vi "control.vi"() -> ()   [LabVIEW 2016]
uses:
  Dynamixel Motor/Public/Motor Operation/Low Level/Baud Setting.ctl
  Program Files (x86)/National Instruments/LabVIEW 2016/examples/Data Communication/Protocols/TCP/TCP Multiple Connections/controls/TCP Multiple Connections State.ctl
  Program Files (x86)/National Instruments/LabVIEW 2016/examples/Data Communication/Protocols/TCP/TCP Multiple Connections/controls/TCP Multiple Connections Data.ctl
  Controller Output.vi
  Dynamixel Motor/Dynamixel Motor.lvlib
panel:
  out "# of Connections 4":i32
  out "# of Connections 3":i32
  out "불리언":bool
  out "불리언 3":bool
  out "# of Connections 2":i32
  out "불리언 2":bool=TRUE
  out "# of Connections":i32
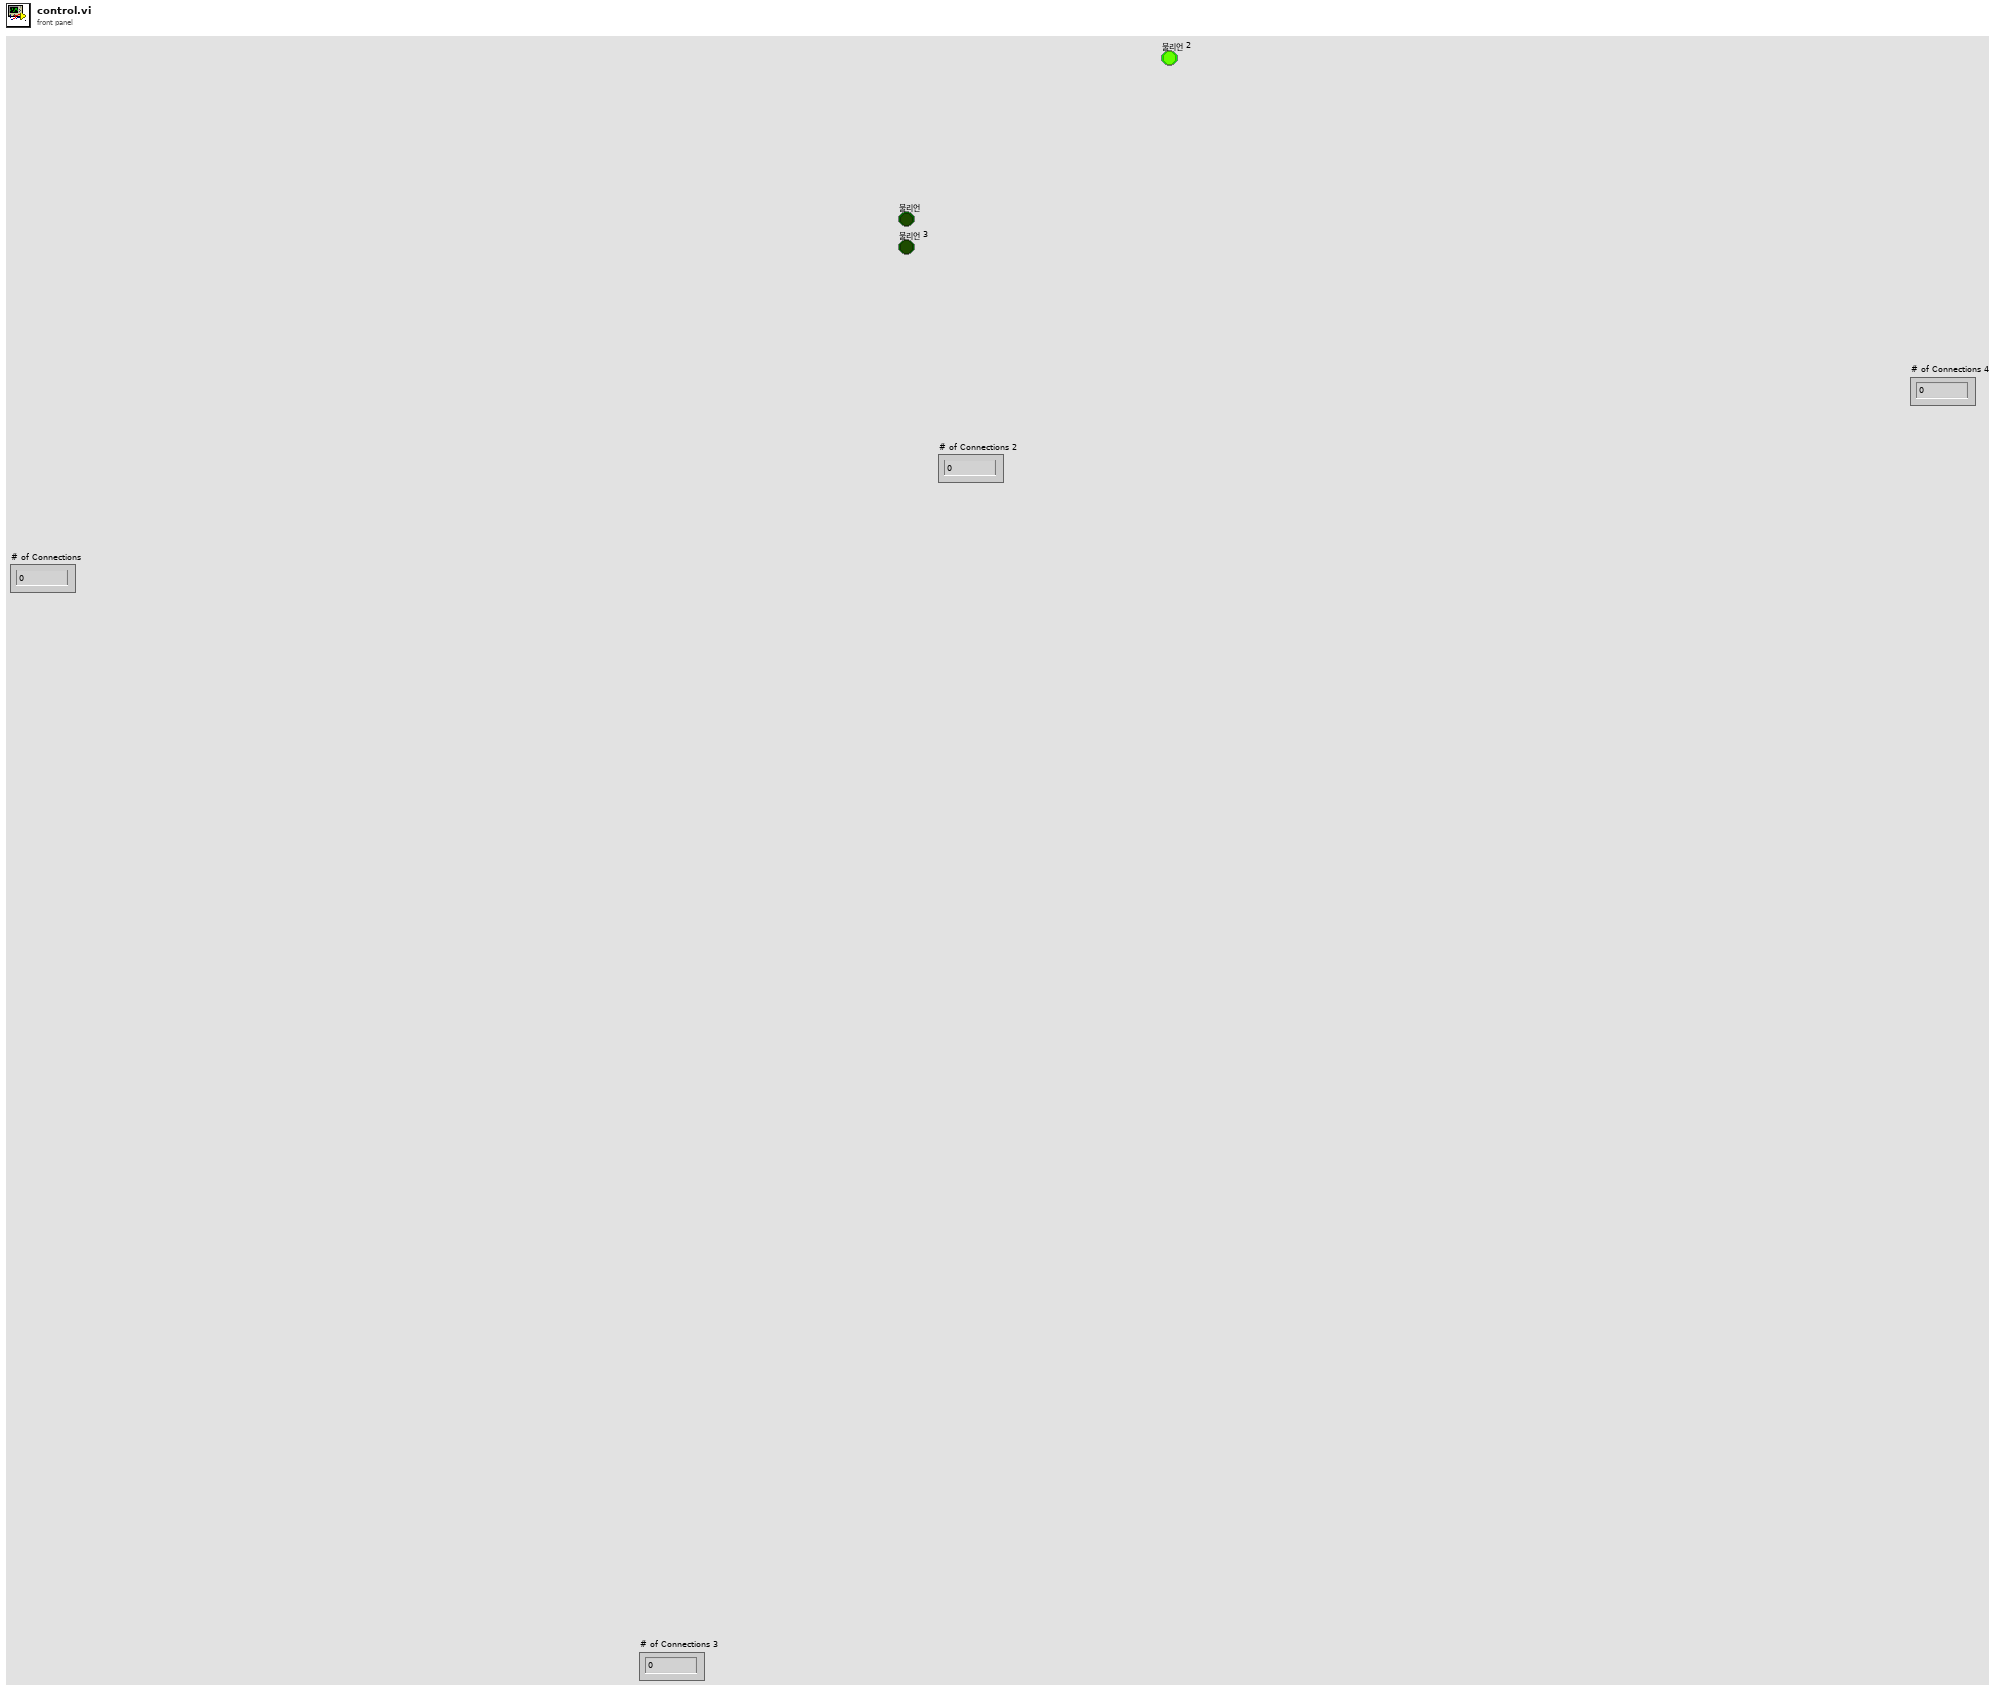
[diagram p1: front panel]
types:
  T1 = typedef "TCP Multiple Connections Data.ctl" = cluster{"Clients":refnum<k5>[], "Listener":refnum<k5>}
  T2 = typedef "TCP Multiple Connections State.ctl" = enum16{"Initialize", "Status Check", "Send Data", "Stop"}
  T3 = typedef "Dynamixel Motor.lvlib/Baud Setting.ctl" = u8
  T4 = typedef "YSH_XBOX360_joystick.ctl" = cluster{"RR":bool, "RL":bool, "RD":bool, "RU":bool, "LR":bool, "LL":bool, "LD":bool, "LU":bool, "Back":bool, "Start":bool, "DPad":dbl, "D Pad":cluster{"0":bool, "45":bool, "90":bool, "135":bool, "180":bool, "215":bool, "270":bool, "315":bool}, "A":bool, "B":bool, "X":bool, "Y":bool, "LB":bool, "RB":bool, "LT":bool, "RT":bool, "Left Joy Push":bool, "Right Joy Push":bool, "Z axis - LT~RT":i32, "Joy1 X-axis":i32, "Joy2 X-axis":i32, "Joy2 Y-axis":i32, "Joy1 Y-axis":i32}
  T5 = enum16{"big-endian, network order", "native, host order", "little-endian"}
  T6 = cluster{"lx":sgl, "ly":sgl, "sla":sgl, "sll":sgl, "rx":sgl, "ry":sgl, "sra":sgl, "srl":sgl, "tl":sgl, "tr":sgl, "bup":sgl, "bdn":sgl, "bl":sgl, "br":sgl, "ba":sgl, "bb":sgl, "bx":sgl, "by":sgl, "back":sgl, "start":sgl, "ls":sgl, "rs":sgl, "lt":sgl, "rt":sgl}
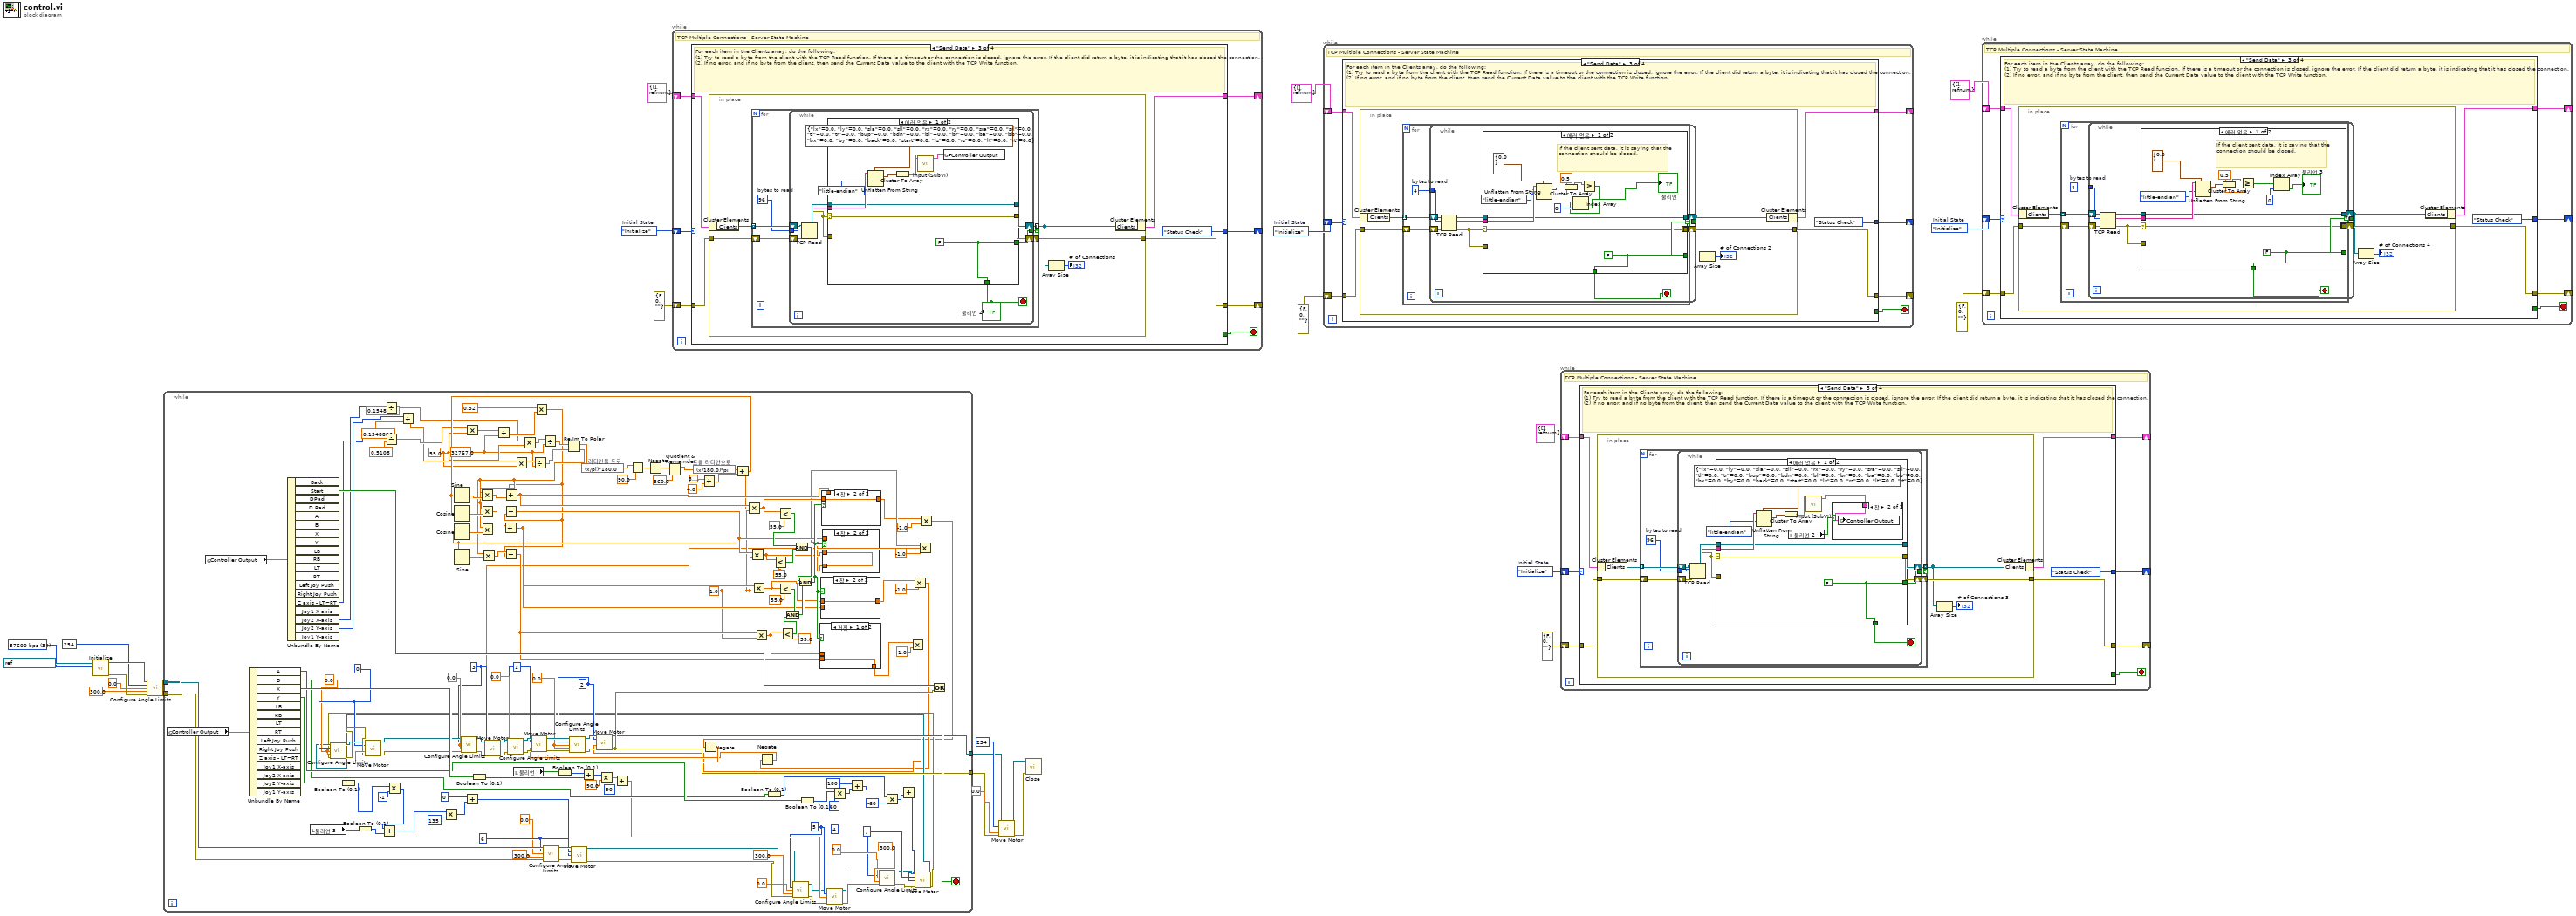
[diagram p0: block diagram]
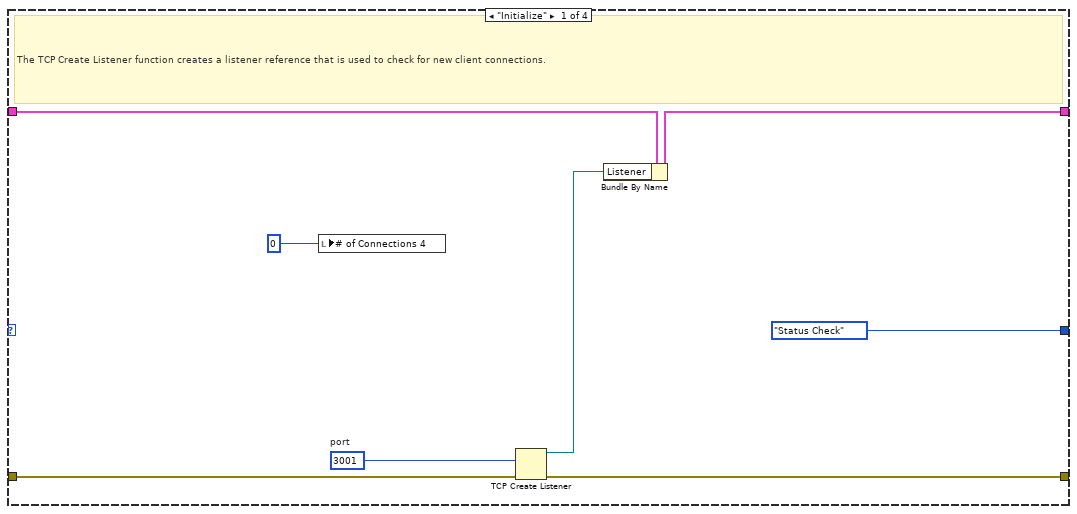
[diagram p2: hidden frame]
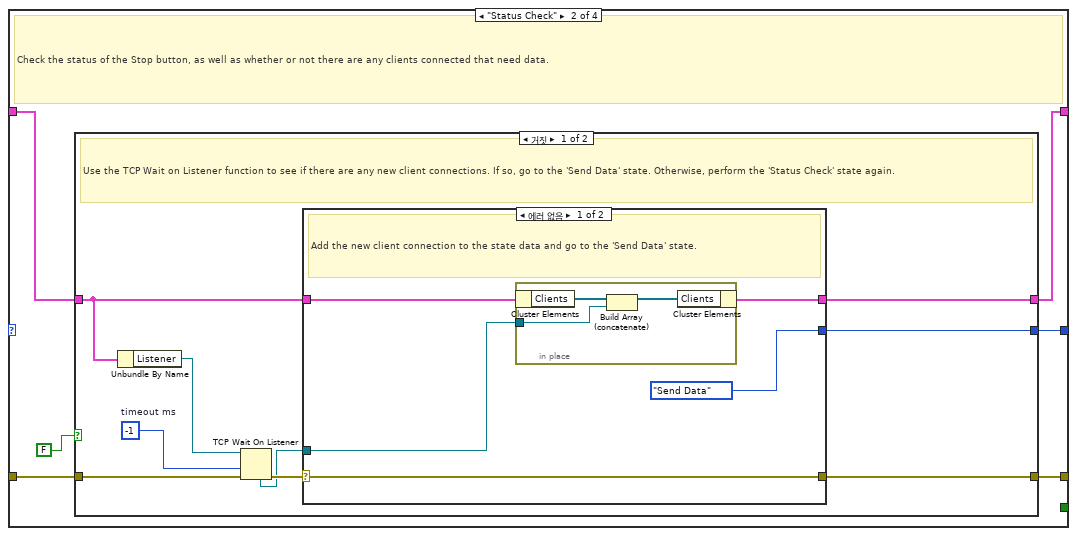
[diagram p3: hidden frame]
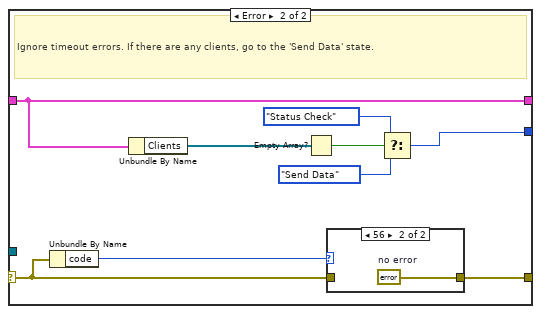
[diagram p4: hidden frame]
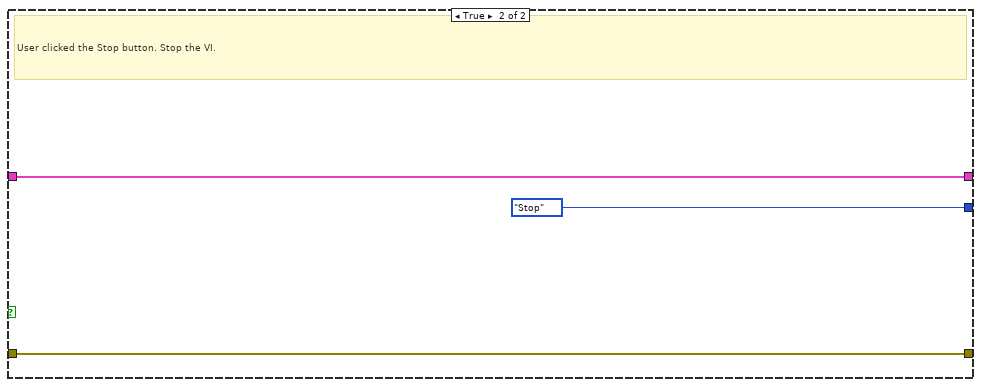
[diagram p6: hidden frame]
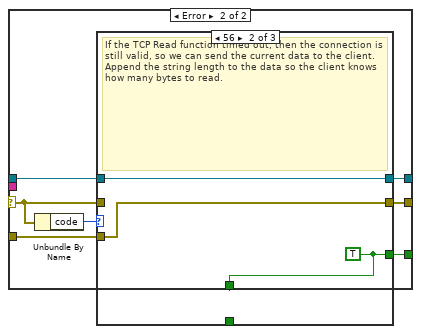
[diagram p7: hidden frame]
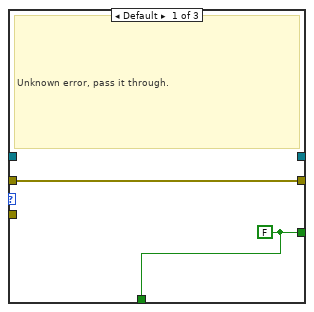
[diagram p8: hidden frame]
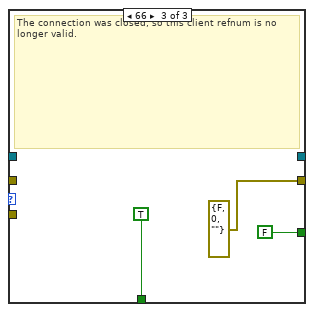
[diagram p9: hidden frame]
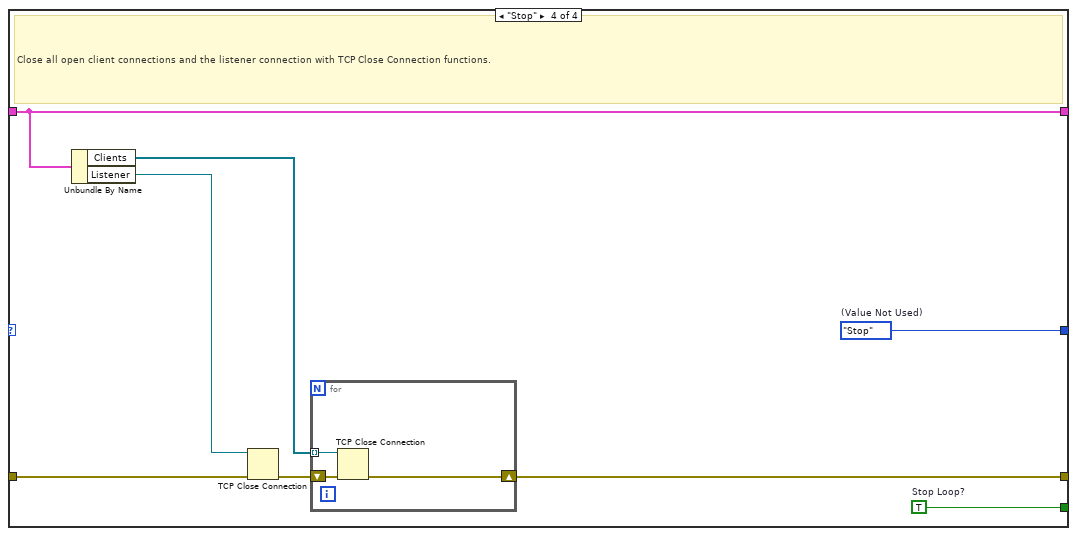
[diagram p10: hidden frame]
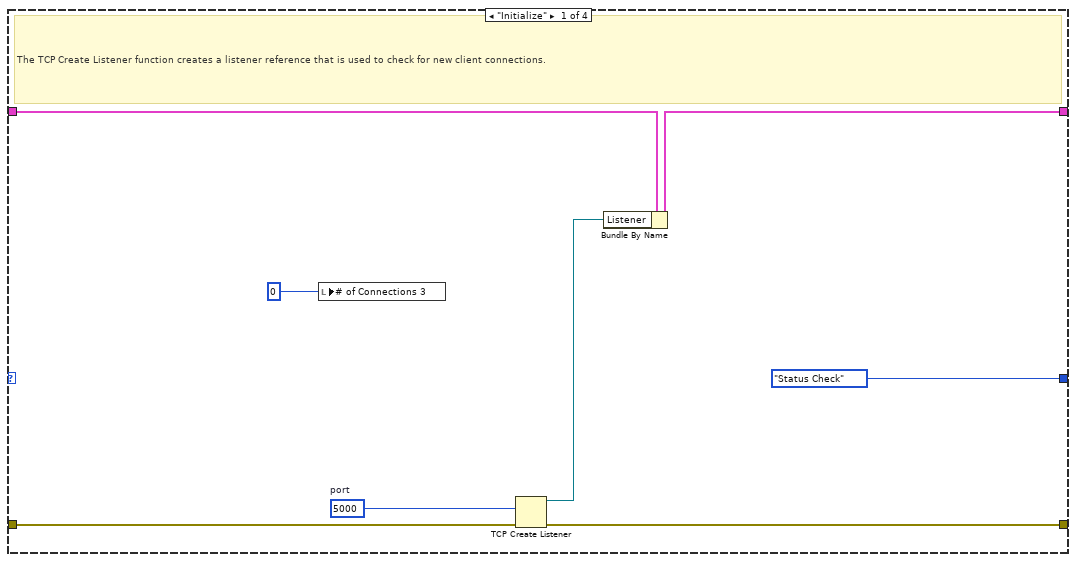
[diagram p15: hidden frame]
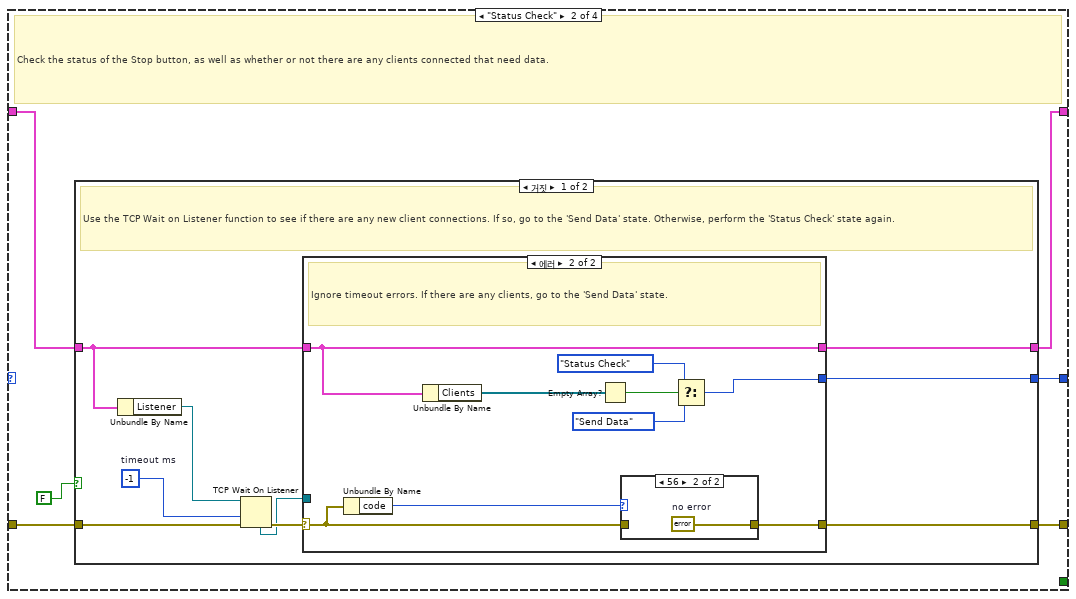
[diagram p16: hidden frame]
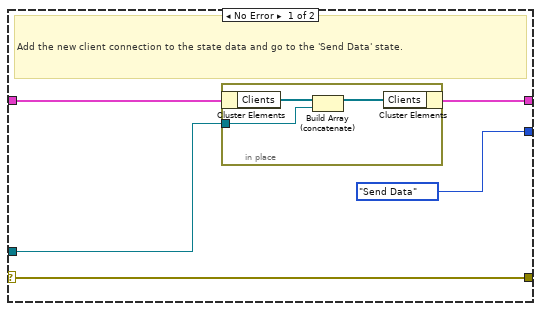
[diagram p17: hidden frame]
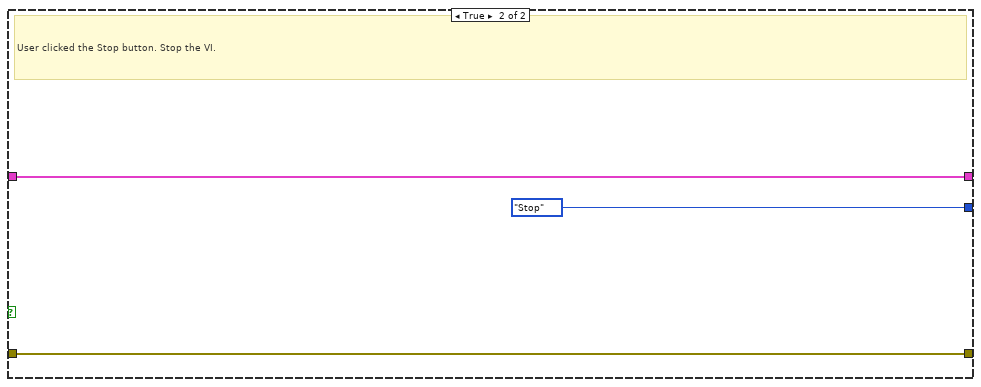
[diagram p19: hidden frame]
diagram:
  w3 = TCP_Multiple_Connections_State."Initialize"  # Initial State
  w17 = T3 34 items=["1,000,000 bps"=1, "500,000 bps"=3, "400,000 bps"=4, "250,000 bps"=7, "200,000 bps"=9, "115200 bps"=16, "57600 bps"=34, "19200 bps"=103, "9600 bps"=207] ("Baud rate (57600 bps) MX")
  w21 = TCP_Multiple_Connections_State."Initialize"  # Initial State
  w24 = TCP_Multiple_Connections_State."Initialize"  # Initial State
  w27 = TCP_Multiple_Connections_State."Initialize"  # Initial State
  n1 = call "Initialize.vi"("Baud rate (57600 bps)"=w17, "VISA resource name"=refnum<visa-resource-name> "ASRL3::INSTR") -> ("error out"=w13:errorcluster, "VISA resource name out"=w16:refnum<visa-resource-name>)  [unwired: 8 in]
  n2 = call "Configure Angle Limits.vi"("VISA resource name"=w16, "Motor ID (0)"=254, "Clockwise Angle Limit (0 deg)"=0.0, "Counter-Clockwise Angle Limit (300 deg)"=300.0, "error in (no error)"=w13) -> ("VISA resource name out"=w15:refnum<visa-resource-name>, "error out"=w14:errorcluster)  [unwired: 9 in]
  n3 = while {
    tunnel: w14 -> [w89]
    tunnel: [w100] -> w6
    tunnel: w15 -> [w91]
    tunnel: [w99] -> w7
    stop <- w126 stop-if-true
    w43 = 32767.0
    w44 = 55.0
    w87 = 6 ("Dynamixel ID AX sorting board 2")
    (unwired) 4 ("Dynamixel ID AX sorting board 2")
    w101 = u8 2 ("Motor ID4")
    w104 = u8 1 ("Motor ID3")
    w121 = u8 0 ("Motor ID1")
    w106 = u8 3 ("Motor ID2")
    w59 = 7 ("Dynamixel ID AX 문 개패 2")
    w49 = 5 ("Dynamixel ID AX sorting board 2")
    w92 = 1.0
    w113 = 0.0
    w105 = 0.0
    w102 = 0.0
    w120 = 0.0
    n4 = global read "Controller Output.vi" "Controller Output"() -> (w138:T4)
    n5 = global read "Controller Output.vi" "Controller Output"() -> (w142:T4)
    n6 = Unbundle By Name(w138) -> ("A"=w140:bool, "B"=w79:bool, "X"=w141:bool, "Y"=w81:bool)  [unwired: 11 out]
    n7 = Unbundle By Name(w142) -> ("Start"=w158:bool, "Z axis - LT~RT"=w71:i32, "Joy2 X-axis"=w73:i32, "Joy2 Y-axis"=w72:i32)  [unwired: 15 out]
    n8 = local read "불리언 3"() -> (w66:bool)
    n9 = Boolean To (0,1)(Boolean=w81) -> (0, 1=w41:i16)
    n10 = Boolean To (0,1)(Boolean=w66) -> (0, 1=w65:i16)
    n11 = Divide(x=w73, y=0.1548886) -> (x/y=w68:dbl)
    n12 = Divide(x=w71, y=0.5108) -> (x/y=w70:dbl)
    n13 = Multiply(x=w41, y=-1) -> (x*y=w40:i32)
    n14 = Add(x=w40, y=w65) -> (x+y=w63:i32)
    n15 = Divide(x=w72, y=0.1548886) -> (x/y=w69:dbl)
    n16 = Multiply(x=w63, y=135) -> (x*y=w83:i32)
    n17 = Multiply(x=w70, y=w44) -> (x*y=w181:dbl)
    n18 = Add(x=0, y=w83) -> (x+y=w82:i32)
    n19 = Boolean To (0,1)(Boolean=w141) -> (0, 1=w132:i16)
    n20 = Divide(x=w181, y=w43) -> (x/y=w97:dbl)
    n21 = Multiply(x=w69, y=w44) -> (x*y=w182:dbl)
    n22 = local read "불리언"() -> (w125:bool)
    n23 = Multiply(x=w68, y=w44) -> (x*y=w183:dbl)
    n24 = Divide(x=w182, y=w43) -> (x/y=w179:dbl)
    n25 = Multiply(x=0.32, y=w97) -> (x*y=w95:dbl)
    n26 = Divide(x=w183, y=w43) -> (x/y=w180:dbl)
    n27 = call "Configure Angle Limits.vi"("VISA resource name"=w91, "Motor ID (0)"=w87, "Clockwise Angle Limit (0 deg)"=0.0, "Counter-Clockwise Angle Limit (300 deg)"=300.0, "error in (no error)"=w89) -> ("VISA resource name out"=w90:refnum<visa-resource-name>, "error out"=w88:errorcluster)  [unwired: 9 in]
    n28 = Boolean To (0,1)(Boolean=w125) -> (0, 1=w131:i16)
    n29 = Re/Im To Polar(2:w179, 3:w180) -> (0:w178:dbl, 1:w163:dbl)
    n30 = call "Move Motor.vi"("VISA resource name"=w90, "Motor ID (0)"=w87, "Goal Position (180 deg)"=w82, "error in (no error)"=w88) -> ("VISA resource name out"=w45:refnum<visa-resource-name>, "error out"=w46:errorcluster)  [unwired: 10 in]
    n31 = Add(x=w131, y=w132) -> (x+y=w130:i16)
    n32 = expression code="(x/pi)*180.0" "라디안을 도로"(w178) -> (w177:dbl)
    n33 = Multiply(x=w130, y=90.0 ("sorting board 각도 input  2")) -> (x*y=w128:dbl)
    n34 = Add(x=w128, y=90) -> (x+y=w52:dbl)
    n35 = Subtract(x=w177, y=90.0) -> (x-y=w176:dbl)
    n36 = Negate(x=w176) -> (-x=w175:dbl)
    n37 = Quotient & Remainder(x=w175, y=360.0) -> (x-y*floor(x/y)=w172:dbl)  [unwired: 1 out]
    n38 = expression code="(x/180.0)*pi" "도를 라디안으로"(w172) -> (w171:dbl)
    n39 = Divide(x=3.141592653589793, y=4.0) -> (x/y=w168:dbl)
    n40 = Add(x=w171, y=w168) -> (x+y=w98:dbl)
    n41 = Sine(x=w98) -> (sin(x)=w167:dbl)
    n42 = Cosine(x=w98) -> (cos(x)=w166:dbl)
    n43 = Cosine(x=w98) -> (cos(x)=w165:dbl)
    n44 = Sine(x=w98) -> (sin(x)=w164:dbl)
    n45 = Multiply(x=w163, y=w167) -> (x*y=w161:dbl)
    n46 = Multiply(x=w163, y=w166) -> (x*y=w160:dbl)
    n47 = Multiply(x=w163, y=w165) -> (x*y=w162:dbl)
    n48 = Multiply(x=w163, y=w164) -> (x*y=w159:dbl)
    n49 = Add(x=w95, y=w162) -> (x+y=w135:dbl)
    n50 = Subtract(x=w160, y=w95) -> (x-y=w136:dbl)
    n51 = Subtract(x=w159, y=w95) -> (x-y=w134:dbl)
    n52 = Add(x=w95, y=w161) -> (x+y=w137:dbl)
    n53 = Multiply(x=w137, y=w92) -> (x*y=w156:dbl)
    n54 = Multiply(x=w136, y=w92) -> (x*y=w145:dbl)
    n55 = Multiply(x=w135, y=w92) -> (x*y=w144:dbl)
    n56 = Multiply(x=w134, y=w92) -> (x*y=w143:dbl)
    n57 = Boolean To (0,1)(Boolean=w79) -> (0, 1=w78:i16)
    n58 = Less?(x=w145, y=55.0) -> (x < y?=w149:bool)
    n59 = Less?(x=w156, y=55.0) -> (x < y?=w155:bool)
    n60 = Less?(x=w144, y=55.0) -> (x < y?=w150:bool)
    n61 = Less?(x=w143, y=55.0) -> (x < y?=w151:bool)
    n62 = And(x=w150, y=w151) -> (x .and. y?=w147:bool)
    n63 = call "Configure Angle Limits.vi"("VISA resource name"=w45, "Motor ID (0)"=w49, "Clockwise Angle Limit (0 deg)"=0.0, "Counter-Clockwise Angle Limit (300 deg)"=300.0, "error in (no error)"=w46) -> ("VISA resource name out"=w48:refnum<visa-resource-name>, "error out"=w47:errorcluster)  [unwired: 9 in]
    n64 = And(x=w155, y=w149) -> (x .and. y?=w148:bool)
    n65 = And(x=w148, y=w147) -> (x .and. y?=w146:bool)
    n66 = Boolean To (0,1)(Boolean=w140) -> (0, 1=w129:i16)
    n67 = case shown="거짓" w146 {
      tunnel: w143 -> [_ w187]
      tunnel: w134 -> [w186 _]
      tunnel: [w186 w187] -> w35
      frame False {
      }
      frame True {
      }
    }
    n68 = case shown="참" w146 {
      tunnel: w144 -> [_ w185]
      tunnel: [w184 w185] -> w33
      tunnel: w135 -> [w184 _]
      frame False {
      }
      frame True {
      }
    }
    n69 = case shown="참" w146 {
      tunnel: w156 -> [_ w191]
      tunnel: [w190 w191] -> w29
      tunnel: w137 -> [w190 _]
      frame False {
      }
      frame True {
      }
    }
    n70 = case shown="참" w146 {
      tunnel: w145 -> [_ w189]
      tunnel: w136 -> [w188 _]
      tunnel: [w188 w189] -> w30
      frame False {
      }
      frame True {
      }
    }
    n71 = call "Move Motor.vi"("VISA resource name"=w48, "Motor ID (0)"=w49, "Goal Position (180 deg)"=w52, "error in (no error)"=w47) -> ("VISA resource name out"=w54:refnum<visa-resource-name>, "error out"=w53:errorcluster)  [unwired: 10 in]
    n72 = Multiply(x=w129, y=60) -> (x*y=w93:i32)
    n73 = Add(x=180, y=w93) -> (x+y=w77:i32)
    n74 = call "Configure Angle Limits.vi"("VISA resource name"=w54, "Motor ID (0)"=w59, "Clockwise Angle Limit (0 deg)"=0.0, "Counter-Clockwise Angle Limit (300 deg)"=300.0, "error in (no error)"=w53) -> ("VISA resource name out"=w58:refnum<visa-resource-name>, "error out"=w60:errorcluster)  [unwired: 9 in]
    n75 = Multiply(x=w78, y=-60) -> (x*y=w76:i32)
    n76 = Add(x=w77, y=w76) -> (x+y=w57:i32)
    n77 = Multiply(x=w35, y=-1.0) -> (x*y=w34:dbl)
    n78 = Multiply(x=w33, y=-1.0) -> (x*y=w32:dbl)
    n79 = Negate(x=w32) -> (-x=w103:dbl)
    n80 = call "Move Motor.vi"("VISA resource name"=w58, "Motor ID (0)"=w59, "Goal Position (180 deg)"=w57, "error in (no error)"=w60) -> ("VISA resource name out"=w56:refnum<visa-resource-name>, "error out"=w55:errorcluster)  [unwired: 10 in]
    n81 = call "Configure Angle Limits.vi"("VISA resource name"=w56, "Motor ID (0)"=w121, "Clockwise Angle Limit (0 deg)"=w120, "Counter-Clockwise Angle Limit (300 deg)"=w120, "error in (no error)"=w55) -> ("VISA resource name out"=w122:refnum<visa-resource-name>, "error out"=w123:errorcluster)  [unwired: 9 in]
    n82 = Multiply(x=w30, y=-1.0) -> (x*y=w31:dbl)
    n83 = Multiply(x=w29, y=-1.0) -> (x*y=w28:dbl)
    n84 = Negate(x=w28) -> (-x=w124:dbl)
    n85 = call "Move Motor.vi"("VISA resource name"=w122, "Motor ID (0)"=w121, "Goal Speed (RPM)"=w124, "error in (no error)"=w123) -> ("VISA resource name out"=w107:refnum<visa-resource-name>, "error out"=w119:errorcluster)  [unwired: 10 in]
    n86 = call "Configure Angle Limits.vi"("VISA resource name"=w107, "Motor ID (0)"=w106, "Clockwise Angle Limit (0 deg)"=w113, "Counter-Clockwise Angle Limit (300 deg)"=w113, "error in (no error)"=w119) -> ("VISA resource name out"=w112:refnum<visa-resource-name>, "error out"=w114:errorcluster)  [unwired: 9 in]
    n87 = call "Move Motor.vi"("VISA resource name"=w112, "Motor ID (0)"=w106, "Goal Speed (RPM)"=w31, "error in (no error)"=w114) -> ("VISA resource name out"=w111:refnum<visa-resource-name>, "error out"=w115:errorcluster)  [unwired: 10 in]
    n88 = call "Configure Angle Limits.vi"("VISA resource name"=w111, "Motor ID (0)"=w104, "Clockwise Angle Limit (0 deg)"=w105, "Counter-Clockwise Angle Limit (300 deg)"=w105, "error in (no error)"=w115) -> ("VISA resource name out"=w110:refnum<visa-resource-name>, "error out"=w116:errorcluster)  [unwired: 9 in]
    n89 = call "Move Motor.vi"("VISA resource name"=w110, "Motor ID (0)"=w104, "Goal Speed (RPM)"=w103, "error in (no error)"=w116) -> ("VISA resource name out"=w109:refnum<visa-resource-name>, "error out"=w117:errorcluster)  [unwired: 10 in]
    n90 = call "Configure Angle Limits.vi"("VISA resource name"=w109, "Motor ID (0)"=w101, "Clockwise Angle Limit (0 deg)"=w102, "Counter-Clockwise Angle Limit (300 deg)"=w102, "error in (no error)"=w117) -> ("VISA resource name out"=w108:refnum<visa-resource-name>, "error out"=w118:errorcluster)  [unwired: 9 in]
    n91 = call "Move Motor.vi"("VISA resource name"=w108, "Motor ID (0)"=w101, "Goal Speed (RPM)"=w34, "error in (no error)"=w118) -> ("VISA resource name out"=w99:refnum<visa-resource-name>, "error out"=w100:errorcluster)  [unwired: 10 in]
    n92 = Or(x=w158, y=w100) -> (x .or. y?=w126:bool)
  }
  n93 = while {
    shift-right: [w197] -> _
    shift-left: w27 -> [w198]
    shift-right: [w195] -> _
    shift-left: T1 {"Clients"=[], "Listener"=refnum} ("Data") -> [w196]
    shift-right: [w193] -> _
    shift-left: errorcluster {"status"=FALSE, "code"=0, "source"=""} ("error constant") -> [w194]
    stop <- w192 stop-if-true
    # "TCP Multiple Connections - Server State Machine"
    n94 = case shown="\"Send Data\"" w198 {
      tunnel: [TCP_Multiple_Connections_State."Status Check" ("States") w212 TCP_Multiple_Connections_State."Status Check" ("States") w296] -> w197
      tunnel: [_ _ _ w303] -> w192
      tunnel: w196 -> [w204 w208 w246 w302]
      tunnel: [w203 w207 w245 w302] -> w195
      tunnel: w194 -> [w206 w211 w248 w301]
      tunnel: [w205 w210 w247 w299] -> w193
      frame "Initialize" {
        w201 = u16 4000  # port
        # "The TCP Create Listener function creates a listener reference that is used to check for new client connections."
        n95 = local write "# of Connections"(0 ("Number of Client Connections")) -> ()
        n96 = TCP Create Listener(8:w206, 10:w201) -> (0:w205:errorcluster, 3:w202:refnum<k5>)  [unwired: 4 out]
        n97 = Bundle By Name(cluster=w204, "Listener"=w202) -> (w203:T1)
      }
      frame "Status Check" {
        # "Check the status of the Stop button, as well as whether or not there are any clients connected that need data."
        n98 = case shown="거짓" FALSE ("Stop") {
          tunnel: [w221 TCP_Multiple_Connections_State."Stop" ("States")] -> w212
          tunnel: w211 -> [w220 w243]
          tunnel: [w213 w243] -> w210
          tunnel: w208 -> [w216 w242]
          tunnel: [w215 w242] -> w207
          frame False {
            w219 = -1  # timeout ms
            # "Use the TCP Wait on Listener function to see if there are any new client connections. If so, go to the 'Send Data' state. Otherwise, perform the 'Status Check' state again."
            n99 = Unbundle By Name(w216) -> ("Listener"=w214:refnum<k5>)
            n100 = TCP Wait On Listener(8:w220, 9:w219, 11:w214) -> (0:w218:errorcluster, 4:w217:refnum<k5>)  [unwired: 4 out]
            n101 = case shown="에러 없음" w218 {
              selector: w218 -> [w224 w238]
              tunnel: [TCP_Multiple_Connections_State."Send Data" ("States") w232] -> w221
              tunnel: w217 -> [w225 _]
              tunnel: w216 -> [w226 w235]
              tunnel: [w223 w235] -> w215
              tunnel: [w224 w236] -> w213
              frame No Error {
                # "Add the new client connection to the state data and go to the 'Send Data' state."
                n102 = in-place {
                  in-place-border: w225 -> [w227]
                  n103 = in-place-cluster #1(w226) -> ("Clients"=w229:refnum<k5>[])
                  n104 = Build Array (concatenate)(w229, w227) -> (w228:refnum<k5>[])
                  n105 = in-place-cluster #1("Clients"=w228) -> (w223:T1)
                }
              }
              frame Error {
                # "Ignore timeout errors. If there are any clients, go to the 'Send Data' state."
                n106 = Unbundle By Name(w238) -> ("code"=w237:i32)
                n107 = Unbundle By Name(w235) -> ("Clients"=w234:refnum<k5>[])
                n108 = Empty Array?(array=w234) -> (empty?=w233:bool)
                n109 = case shown="56" w237 {
                  tunnel: w238 -> [w239 _]
                  tunnel: [w239 w240] -> w236
                  frame Default {
                  }
                  frame 56 {
                    w240 = errorcluster {"status"=FALSE, "code"=0, "source"=""}  # no error
                  }
                }
                n110 = Select(t=TCP_Multiple_Connections_State."Status Check" ("States"), s=w233, f=TCP_Multiple_Connections_State."Send Data" ("States")) -> (s? t:f=w232:T2)
              }
            }
          }
          frame True {
            # "User clicked the Stop button. Stop the VI."
          }
        }
      }
      frame "Send Data" {
        # "For each item in the Clients array, do the following:\n(1) Try to read a byte from the client with the TCP Read function. If there is a timeout or the connection is closed, ignore the error. If the client did return a byte, it is indicating that it has closed the connection.\n(2) If no error, and if no byte from the client, then send the Current Data value to the client with the TCP Write function."
        n111 = in-place {
          in-place-border: w248 -> [w253]
          in-place-border: [w252] -> w247
          n112 = in-place-cluster #2(w246) -> ("Clients"=w250:refnum<k5>[])
          n113 = for {
            tunnel: w250 -> [w259] mode=indexing
            shift-right: [w255] -> w252
            shift-left: w253 -> [w254]
            tunnel: [w257] -> w249 mode=indexing if=w256
            w258 = 96  # bytes to read
            n114 = while {
              tunnel: w258 -> [w267]
              tunnel: [w264] -> w256
              shift-right: [w265] -> w257
              shift-left: w259 -> [w269]
              shift-right: [w261] -> w255
              shift-left: w254 -> [w263]
              stop <- w260 stop-if-true
              n115 = TCP Read(connection ID=w269, bytes to read=w267, error in (no error)=w263) -> (connection ID out=w268:refnum<k5>, data out=w266:string, error out=w262:errorcluster)  [unwired: 1 in, 1 out]
              n116 = case shown="에러 없음" w262 {
                selector: w262 -> [w271 w285]
                tunnel: w268 -> [w277 w284]
                tunnel: w266 -> [w278 _]
                tunnel: [w277 w282] -> w265
                tunnel: [w270 w283] -> w264
                tunnel: [w271 w281] -> w261
                tunnel: w262 -> [_ w280]
                tunnel: [w270 w279] -> w260
                frame No Error {
                  w270 = FALSE
                  # "If the client sent data, it is saying that the connection should be closed."
                  n117 = Unflatten From String(type=T6 {"lx"=0.0, "ly"=0.0, "sla"=0.0, "sll"=0.0, "rx"=0.0, "ry"=0.0, "sra"=0.0, "srl"=0.0, "tl"=0.0, "tr"=0.0, "bup"=0.0, "bdn"=0.0, "bl"=0.0, "br"=0.0, "ba"=0.0, "bb"=0.0, "bx"=0.0, "by"=0.0, "back"=0.0, "start"=0.0, "ls"=0.0, "rs"=0.0, "lt"=0.0, "rt"=0.0}, binary string=w278, byte order (0:big-endian, network order)=T5."little-endian") -> (value=w276:T6)  [unwired: 2 in, 2 out]
                  n118 = Cluster To Array(cluster=w276) -> (array=w273:sgl[])
                  n119 = call "input (SubVI).vi"("Controller_NUC"=w273) -> ("Controller Input"=w272:T4)  [unwired: 10 in]
                  n120 = global write "Controller Output.vi" "Controller Output"(w272) -> ()
                }
                frame Error {
                  # "Ignore connection closed and timeout errors"
                  n121 = Unbundle By Name(w285) -> ("code"=w286:i32)
                  n122 = case shown="66" w286 {
                    tunnel: w285 -> [w288 _ _]
                    tunnel: [w288 w290 errorcluster {"status"=FALSE, "code"=0, "source"=""} ("error constant")] -> w281
                    tunnel: w284 -> [_ w291 _]
                    tunnel: [w287 TRUE FALSE] -> w283
                    tunnel: [_ w291 _] -> w282
                    tunnel: w280 -> [_ w290 _]
                    tunnel: [w287 TRUE TRUE] -> w279
                    frame Default {
                      w287 = FALSE
                      # "Unknown error, pass it through."
                    }
                    frame 56 {
                      # "If the TCP Read function timed out, then the connection is still valid, so we can send the current data to the client. Append the string length to the data so the client knows how many bytes to read."
                    }
                    frame 66 {
                      # "The connection was closed, so this client refnum is no longer valid."
                    }
                  }
                }
              }
              "불리언 2" <- w260
            }
          }
          n123 = Array Size(array=w249) -> (size(s)=→"# of Connections":i32)
          n124 = in-place-cluster #2("Clients"=w249) -> (w245:T1)
        }
      }
      frame "Stop" {
        w296 = TCP_Multiple_Connections_State."Stop"  # (Value Not Used)
        w303 = TRUE  # Stop Loop?
        # "Close all open client connections and the listener connection with TCP Close Connection functions."
        n125 = Unbundle By Name(w302) -> ("Clients"=w300:refnum<k5>[], "Listener"=w297:refnum<k5>)
        n126 = TCP Close Connection(connection ID=w297, error in (no error)=w301) -> (error out=w298:errorcluster)  [unwired: 1 in, 1 out]
        n127 = for {
          shift-right: [w305] -> w299
          shift-left: w298 -> [w306]
          tunnel: w300 -> [w304] mode=indexing
          n128 = TCP Close Connection(connection ID=w304, error in (no error)=w306) -> (error out=w305:errorcluster)  [unwired: 1 in, 1 out]
        }
      }
    }
  }
  n129 = call "Move Motor.vi"("VISA resource name"=w7, "Motor ID (0)"=254, "Goal Speed (RPM)"=0.0, "error in (no error)"=w6) -> ("VISA resource name out"=w5:refnum<visa-resource-name>, "error out"=w4:errorcluster)  [unwired: 10 in]
  n130 = call "Close.vi"("error in (no error)"=w4, "VISA resource name"=w5) -> ()  [unwired: 9 in, 1 out]
  n131 = while {
    shift-right: [w312] -> _
    shift-left: w24 -> [w313]
    shift-right: [w310] -> _
    shift-left: T1 {"Clients"=[], "Listener"=refnum} ("Data") -> [w311]
    shift-right: [w308] -> _
    shift-left: errorcluster {"status"=FALSE, "code"=0, "source"=""} ("error constant") -> [w309]
    stop <- w307 stop-if-true
    # "TCP Multiple Connections - Server State Machine"
    n132 = case shown="\"Send Data\"" w313 {
      tunnel: [TCP_Multiple_Connections_State."Status Check" ("States") w327 TCP_Multiple_Connections_State."Status Check" ("States") w413] -> w312
      tunnel: [_ _ _ w420] -> w307
      tunnel: w311 -> [w319 w323 w361 w419]
      tunnel: [w318 w322 w360 w419] -> w310
      tunnel: w309 -> [w321 w326 w363 w418]
      tunnel: [w320 w325 w362 w416] -> w308
      frame "Initialize" {
        w316 = u16 3000  # port
        # "The TCP Create Listener function creates a listener reference that is used to check for new client connections."
        n133 = local write "# of Connections 2"(0 ("Number of Client Connections")) -> ()
        n134 = TCP Create Listener(8:w321, 10:w316) -> (0:w320:errorcluster, 3:w317:refnum<k5>)  [unwired: 4 out]
        n135 = Bundle By Name(cluster=w319, "Listener"=w317) -> (w318:T1)
      }
      frame "Status Check" {
        # "Check the status of the Stop button, as well as whether or not there are any clients connected that need data."
        n136 = case shown="거짓" FALSE ("Stop 2") {
          tunnel: [w336 TCP_Multiple_Connections_State."Stop" ("States")] -> w327
          tunnel: w326 -> [w335 w358]
          tunnel: [w328 w358] -> w325
          tunnel: w323 -> [w331 w357]
          tunnel: [w330 w357] -> w322
          frame False {
            w334 = -1  # timeout ms
            # "Use the TCP Wait on Listener function to see if there are any new client connections. If so, go to the 'Send Data' state. Otherwise, perform the 'Status Check' state again."
            n137 = Unbundle By Name(w331) -> ("Listener"=w329:refnum<k5>)
            n138 = TCP Wait On Listener(8:w335, 9:w334, 11:w329) -> (0:w333:errorcluster, 4:w332:refnum<k5>)  [unwired: 4 out]
            n139 = case shown="에러 없음" w333 {
              selector: w333 -> [w339 w353]
              tunnel: [TCP_Multiple_Connections_State."Send Data" ("States") w347] -> w336
              tunnel: w332 -> [w340 _]
              tunnel: w331 -> [w341 w350]
              tunnel: [w338 w350] -> w330
              tunnel: [w339 w351] -> w328
              frame No Error {
                # "Add the new client connection to the state data and go to the 'Send Data' state."
                n140 = in-place {
                  in-place-border: w340 -> [w342]
                  n141 = in-place-cluster #3(w341) -> ("Clients"=w344:refnum<k5>[])
                  n142 = Build Array (concatenate)(w344, w342) -> (w343:refnum<k5>[])
                  n143 = in-place-cluster #3("Clients"=w343) -> (w338:T1)
                }
              }
              frame Error {
                # "Ignore timeout errors. If there are any clients, go to the 'Send Data' state."
                n144 = Unbundle By Name(w353) -> ("code"=w352:i32)
                n145 = Unbundle By Name(w350) -> ("Clients"=w349:refnum<k5>[])
                n146 = Empty Array?(array=w349) -> (empty?=w348:bool)
                n147 = case shown="56" w352 {
                  tunnel: w353 -> [w354 _]
                  tunnel: [w354 w355] -> w351
                  frame Default {
                  }
                  frame 56 {
                    w355 = errorcluster {"status"=FALSE, "code"=0, "source"=""}  # no error
                  }
                }
                n148 = Select(t=TCP_Multiple_Connections_State."Status Check" ("States"), s=w348, f=TCP_Multiple_Connections_State."Send Data" ("States")) -> (s? t:f=w347:T2)
              }
            }
          }
          frame True {
            # "User clicked the Stop button. Stop the VI."
          }
        }
      }
      frame "Send Data" {
        # "For each item in the Clients array, do the following:\n(1) Try to read a byte from the client with the TCP Read function. If there is a timeout or the connection is closed, ignore the error. If the client did return a byte, it is indicating that it has closed the connection.\n(2) If no error, and if no byte from the client, then send the Current Data value to the client with the TCP Write function."
        n149 = in-place {
          in-place-border: w363 -> [w368]
          in-place-border: [w367] -> w362
          n150 = in-place-cluster #4(w361) -> ("Clients"=w365:refnum<k5>[])
          n151 = for {
            tunnel: w365 -> [w374] mode=indexing
            shift-right: [w370] -> w367
            shift-left: w368 -> [w369]
            tunnel: [w372] -> w364 mode=indexing if=w371
            w373 = 4  # bytes to read
            n152 = while {
              tunnel: w373 -> [w382]
              tunnel: [w379] -> w371
              shift-right: [w380] -> w372
              shift-left: w374 -> [w384]
              shift-right: [w377] -> w370
              shift-left: w369 -> [w378]
              stop <- w376 stop-if-true
              n153 = TCP Read(connection ID=w384, bytes to read=w382, error in (no error)=w378) -> (connection ID out=w383:refnum<k5>, data out=w381:string, error out=w375:errorcluster)  [unwired: 1 in, 1 out]
              n154 = case shown="에러 없음" w375 {
                selector: w375 -> [w388 w403]
                tunnel: w383 -> [w395 w401]
                tunnel: w381 -> [w396 _]
                tunnel: [w395 w399] -> w380
                tunnel: [w387 w400] -> w379
                tunnel: [w388 w398] -> w377
                tunnel: w375 -> [_ w402]
                tunnel: [w387 w397] -> w376
                frame No Error {
                  w387 = FALSE
                  # "If the client sent data, it is saying that the connection should be closed."
                  # "If the client sent data, it is saying that the connection should be closed."
                  n155 = Unflatten From String(type=cluster{"bx":sgl} {"bx"=0.0}, binary string=w396, byte order (0:big-endian, network order)=T5."little-endian") -> (value=w393:cluster{"bx":sgl})  [unwired: 2 in, 2 out]
                  n156 = Cluster To Array(cluster=w393) -> (array=w390:sgl[])
                  n157 = Greater Or Equal?(x=w390, y=0.5) -> (x >= y?=w385:bool[])
                  n158 = Index Array(array=w385, index=0) -> (element=→"불리언":bool)
                }
                frame Error {
                  # "Ignore connection closed and timeout errors"
                  n159 = Unbundle By Name(w403) -> ("code"=w404:i32)
                  n160 = case shown="56" w404 {
                    tunnel: w403 -> [w406 _ _]
                    tunnel: [w406 w409 errorcluster {"status"=FALSE, "code"=0, "source"=""} ("error constant")] -> w398
                    tunnel: w402 -> [_ w409 _]
                    tunnel: w401 -> [_ w408 _]
                    tunnel: [w405 w407 FALSE] -> w400
                    tunnel: [_ w408 _] -> w399
                    tunnel: [w405 w407 TRUE] -> w397
                    frame Default {
                      w405 = FALSE
                      # "Unknown error, pass it through."
                    }
                    frame 56 {
                      w407 = TRUE
                      # "If the TCP Read function timed out, then the connection is still valid, so we can send the current data to the client. Append the string length to the data so the client knows how many bytes to read."
                    }
                    frame 66 {
                      # "The connection was closed, so this client refnum is no longer valid."
                    }
                  }
                }
              }
            }
          }
          n161 = Array Size(array=w364) -> (size(s)=→"# of Connections 2":i32)
          n162 = in-place-cluster #4("Clients"=w364) -> (w360:T1)
        }
      }
      frame "Stop" {
        w413 = TCP_Multiple_Connections_State."Stop"  # (Value Not Used)
        w420 = TRUE  # Stop Loop?
        # "Close all open client connections and the listener connection with TCP Close Connection functions."
        n163 = Unbundle By Name(w419) -> ("Clients"=w417:refnum<k5>[], "Listener"=w414:refnum<k5>)
        n164 = TCP Close Connection(connection ID=w414, error in (no error)=w418) -> (error out=w415:errorcluster)  [unwired: 1 in, 1 out]
        n165 = for {
          shift-right: [w422] -> w416
          shift-left: w415 -> [w423]
          tunnel: w417 -> [w421] mode=indexing
          n166 = TCP Close Connection(connection ID=w421, error in (no error)=w423) -> (error out=w422:errorcluster)  [unwired: 1 in, 1 out]
        }
      }
    }
  }
  n167 = while {
    shift-right: [w429] -> _
    shift-left: w21 -> [w430]
    shift-right: [w427] -> _
    shift-left: T1 {"Clients"=[], "Listener"=refnum} ("Data") -> [w428]
    shift-right: [w425] -> _
    shift-left: errorcluster {"status"=FALSE, "code"=0, "source"=""} ("error constant") -> [w426]
    stop <- w424 stop-if-true
    # "TCP Multiple Connections - Server State Machine"
    n168 = case shown="\"Send Data\"" w430 {
      tunnel: [TCP_Multiple_Connections_State."Status Check" ("States") w444 TCP_Multiple_Connections_State."Status Check" ("States") w530] -> w429
      tunnel: [_ _ _ w537] -> w424
      tunnel: w428 -> [w436 w440 w478 w536]
      tunnel: [w435 w439 w477 w536] -> w427
      tunnel: w426 -> [w438 w443 w480 w535]
      tunnel: [w437 w442 w479 w533] -> w425
      frame "Initialize" {
        w433 = u16 5000  # port
        # "The TCP Create Listener function creates a listener reference that is used to check for new client connections."
        n169 = local write "# of Connections 3"(0 ("Number of Client Connections")) -> ()
        n170 = TCP Create Listener(8:w438, 10:w433) -> (0:w437:errorcluster, 3:w434:refnum<k5>)  [unwired: 4 out]
        n171 = Bundle By Name(cluster=w436, "Listener"=w434) -> (w435:T1)
      }
      frame "Status Check" {
        # "Check the status of the Stop button, as well as whether or not there are any clients connected that need data."
        n172 = case shown="거짓" FALSE ("Stop") {
          tunnel: [w453 TCP_Multiple_Connections_State."Stop" ("States")] -> w444
          tunnel: w443 -> [w452 w475]
          tunnel: [w445 w475] -> w442
          tunnel: w440 -> [w448 w474]
          tunnel: [w447 w474] -> w439
          frame False {
            w451 = -1  # timeout ms
            # "Use the TCP Wait on Listener function to see if there are any new client connections. If so, go to the 'Send Data' state. Otherwise, perform the 'Status Check' state again."
            n173 = Unbundle By Name(w448) -> ("Listener"=w446:refnum<k5>)
            n174 = TCP Wait On Listener(8:w452, 9:w451, 11:w446) -> (0:w450:errorcluster, 4:w449:refnum<k5>)  [unwired: 4 out]
            n175 = case shown="에러" w450 {
              selector: w450 -> [w456 w470]
              tunnel: [TCP_Multiple_Connections_State."Send Data" ("States") w464] -> w453
              tunnel: w449 -> [w457 _]
              tunnel: w448 -> [w458 w467]
              tunnel: [w455 w467] -> w447
              tunnel: [w456 w468] -> w445
              frame No Error {
                # "Add the new client connection to the state data and go to the 'Send Data' state."
                n176 = in-place {
                  in-place-border: w457 -> [w459]
                  n177 = in-place-cluster #5(w458) -> ("Clients"=w461:refnum<k5>[])
                  n178 = Build Array (concatenate)(w461, w459) -> (w460:refnum<k5>[])
                  n179 = in-place-cluster #5("Clients"=w460) -> (w455:T1)
                }
              }
              frame Error {
                # "Ignore timeout errors. If there are any clients, go to the 'Send Data' state."
                n180 = Unbundle By Name(w470) -> ("code"=w469:i32)
                n181 = Unbundle By Name(w467) -> ("Clients"=w466:refnum<k5>[])
                n182 = Empty Array?(array=w466) -> (empty?=w465:bool)
                n183 = case shown="56" w469 {
                  tunnel: w470 -> [w471 _]
                  tunnel: [w471 w472] -> w468
                  frame Default {
                  }
                  frame 56 {
                    w472 = errorcluster {"status"=FALSE, "code"=0, "source"=""}  # no error
                  }
                }
                n184 = Select(t=TCP_Multiple_Connections_State."Status Check" ("States"), s=w465, f=TCP_Multiple_Connections_State."Send Data" ("States")) -> (s? t:f=w464:T2)
              }
            }
          }
          frame True {
            # "User clicked the Stop button. Stop the VI."
          }
        }
      }
      frame "Send Data" {
        # "For each item in the Clients array, do the following:\n(1) Try to read a byte from the client with the TCP Read function. If there is a timeout or the connection is closed, ignore the error. If the client did return a byte, it is indicating that it has closed the connection.\n(2) If no error, and if no byte from the client, then send the Current Data value to the client with the TCP Write function."
        n185 = in-place {
          in-place-border: w480 -> [w485]
          in-place-border: [w484] -> w479
          n186 = in-place-cluster #6(w478) -> ("Clients"=w482:refnum<k5>[])
          n187 = for {
            tunnel: w482 -> [w491] mode=indexing
            shift-right: [w487] -> w484
            shift-left: w485 -> [w486]
            tunnel: [w489] -> w481 mode=indexing if=w488
            w490 = 96  # bytes to read
            n188 = while {
              tunnel: w490 -> [w499]
              tunnel: [w496] -> w488
              shift-right: [w497] -> w489
              shift-left: w491 -> [w501]
              shift-right: [w493] -> w487
              shift-left: w486 -> [w495]
              stop <- w492 stop-if-true
              n189 = TCP Read(connection ID=w501, bytes to read=w499, error in (no error)=w495) -> (connection ID out=w500:refnum<k5>, data out=w498:string, error out=w494:errorcluster)  [unwired: 1 in, 1 out]
              n190 = case shown="에러 없음" w494 {
                selector: w494 -> [w505 w519]
                tunnel: w500 -> [w510 w518]
                tunnel: w498 -> [w511 _]
                tunnel: [w510 w516] -> w497
                tunnel: [w504 w517] -> w496
                tunnel: [w505 w515] -> w493
                tunnel: w494 -> [_ w514]
                tunnel: [w504 w513] -> w492
                frame No Error {
                  w504 = FALSE
                  # "If the client sent data, it is saying that the connection should be closed."
                  n191 = Unflatten From String(type=T6 {"lx"=0.0, "ly"=0.0, "sla"=0.0, "sll"=0.0, "rx"=0.0, "ry"=0.0, "sra"=0.0, "srl"=0.0, "tl"=0.0, "tr"=0.0, "bup"=0.0, "bdn"=0.0, "bl"=0.0, "br"=0.0, "ba"=0.0, "bb"=0.0, "bx"=0.0, "by"=0.0, "back"=0.0, "start"=0.0, "ls"=0.0, "rs"=0.0, "lt"=0.0, "rt"=0.0}, binary string=w511, byte order (0:big-endian, network order)=T5."little-endian") -> (value=w509:T6)  [unwired: 2 in, 2 out]
                  n192 = Cluster To Array(cluster=w509) -> (array=w506:sgl[])
                  n193 = local read "불리언 2"() -> (w502:bool)
                  n194 = call "input (SubVI).vi"("Controller_NUC"=w506) -> ("Controller Input"=w503:T4)  [unwired: 10 in]
                  n195 = case shown="참" w502 {
                    tunnel: w503 -> [_ w512]
                    frame False {
                    }
                    frame True {
                      n196 = global write "Controller Output.vi" "Controller Output"(w512) -> ()
                    }
                  }
                }
                frame Error {
                  # "Ignore connection closed and timeout errors"
                  n197 = Unbundle By Name(w519) -> ("code"=w520:i32)
                  n198 = case shown="66" w520 {
                    tunnel: w519 -> [w522 _ _]
                    tunnel: [w522 w524 errorcluster {"status"=FALSE, "code"=0, "source"=""} ("error constant")] -> w515
                    tunnel: w518 -> [_ w525 _]
                    tunnel: [w521 TRUE FALSE] -> w517
                    tunnel: [_ w525 _] -> w516
                    tunnel: w514 -> [_ w524 _]
                    tunnel: [w521 TRUE TRUE] -> w513
                    frame Default {
                      w521 = FALSE
                      # "Unknown error, pass it through."
                    }
                    frame 56 {
                      # "If the TCP Read function timed out, then the connection is still valid, so we can send the current data to the client. Append the string length to the data so the client knows how many bytes to read."
                    }
                    frame 66 {
                      # "The connection was closed, so this client refnum is no longer valid."
                    }
                  }
                }
              }
            }
          }
          n199 = Array Size(array=w481) -> (size(s)=→"# of Connections 3":i32)
          n200 = in-place-cluster #6("Clients"=w481) -> (w477:T1)
        }
      }
      frame "Stop" {
        w530 = TCP_Multiple_Connections_State."Stop"  # (Value Not Used)
        w537 = TRUE  # Stop Loop?
        # "Close all open client connections and the listener connection with TCP Close Connection functions."
        n201 = Unbundle By Name(w536) -> ("Clients"=w534:refnum<k5>[], "Listener"=w531:refnum<k5>)
        n202 = TCP Close Connection(connection ID=w531, error in (no error)=w535) -> (error out=w532:errorcluster)  [unwired: 1 in, 1 out]
        n203 = for {
          shift-right: [w539] -> w533
          shift-left: w532 -> [w540]
          tunnel: w534 -> [w538] mode=indexing
          n204 = TCP Close Connection(connection ID=w538, error in (no error)=w540) -> (error out=w539:errorcluster)  [unwired: 1 in, 1 out]
        }
      }
    }
  }
  n205 = while {
    shift-right: [w546] -> _
    shift-left: w3 -> [w547]
    shift-right: [w544] -> _
    shift-left: T1 {"Clients"=[], "Listener"=refnum} ("Data") -> [w545]
    shift-right: [w542] -> _
    shift-left: errorcluster {"status"=FALSE, "code"=0, "source"=""} ("error constant") -> [w543]
    stop <- w541 stop-if-true
    # "TCP Multiple Connections - Server State Machine"
    n206 = case shown="\"Send Data\"" w547 {
      tunnel: [TCP_Multiple_Connections_State."Status Check" ("States") w561 TCP_Multiple_Connections_State."Status Check" ("States") w647] -> w546
      tunnel: [_ _ _ w654] -> w541
      tunnel: w545 -> [w553 w557 w595 w653]
      tunnel: [w552 w556 w594 w653] -> w544
      tunnel: w543 -> [w555 w560 w597 w652]
      tunnel: [w554 w559 w596 w650] -> w542
      frame "Initialize" {
        w550 = u16 3001  # port
        # "The TCP Create Listener function creates a listener reference that is used to check for new client connections."
        n207 = local write "# of Connections 4"(0 ("Number of Client Connections")) -> ()
        n208 = TCP Create Listener(8:w555, 10:w550) -> (0:w554:errorcluster, 3:w551:refnum<k5>)  [unwired: 4 out]
        n209 = Bundle By Name(cluster=w553, "Listener"=w551) -> (w552:T1)
      }
      frame "Status Check" {
        # "Check the status of the Stop button, as well as whether or not there are any clients connected that need data."
        n210 = case shown="거짓" FALSE ("Stop 2") {
          tunnel: [w570 TCP_Multiple_Connections_State."Stop" ("States")] -> w561
          tunnel: w560 -> [w569 w592]
          tunnel: [w562 w592] -> w559
          tunnel: w557 -> [w565 w591]
          tunnel: [w564 w591] -> w556
          frame False {
            w568 = -1  # timeout ms
            # "Use the TCP Wait on Listener function to see if there are any new client connections. If so, go to the 'Send Data' state. Otherwise, perform the 'Status Check' state again."
            n211 = Unbundle By Name(w565) -> ("Listener"=w563:refnum<k5>)
            n212 = TCP Wait On Listener(8:w569, 9:w568, 11:w563) -> (0:w567:errorcluster, 4:w566:refnum<k5>)  [unwired: 4 out]
            n213 = case shown="에러 없음" w567 {
              selector: w567 -> [w573 w587]
              tunnel: [TCP_Multiple_Connections_State."Send Data" ("States") w581] -> w570
              tunnel: w566 -> [w574 _]
              tunnel: w565 -> [w575 w584]
              tunnel: [w572 w584] -> w564
              tunnel: [w573 w585] -> w562
              frame No Error {
                # "Add the new client connection to the state data and go to the 'Send Data' state."
                n214 = in-place {
                  in-place-border: w574 -> [w576]
                  n215 = in-place-cluster #7(w575) -> ("Clients"=w578:refnum<k5>[])
                  n216 = Build Array (concatenate)(w578, w576) -> (w577:refnum<k5>[])
                  n217 = in-place-cluster #7("Clients"=w577) -> (w572:T1)
                }
              }
              frame Error {
                # "Ignore timeout errors. If there are any clients, go to the 'Send Data' state."
                n218 = Unbundle By Name(w587) -> ("code"=w586:i32)
                n219 = Unbundle By Name(w584) -> ("Clients"=w583:refnum<k5>[])
                n220 = Empty Array?(array=w583) -> (empty?=w582:bool)
                n221 = case shown="56" w586 {
                  tunnel: w587 -> [w588 _]
                  tunnel: [w588 w589] -> w585
                  frame Default {
                  }
                  frame 56 {
                    w589 = errorcluster {"status"=FALSE, "code"=0, "source"=""}  # no error
                  }
                }
                n222 = Select(t=TCP_Multiple_Connections_State."Status Check" ("States"), s=w582, f=TCP_Multiple_Connections_State."Send Data" ("States")) -> (s? t:f=w581:T2)
              }
            }
          }
          frame True {
            # "User clicked the Stop button. Stop the VI."
          }
        }
      }
      frame "Send Data" {
        # "For each item in the Clients array, do the following:\n(1) Try to read a byte from the client with the TCP Read function. If there is a timeout or the connection is closed, ignore the error. If the client did return a byte, it is indicating that it has closed the connection.\n(2) If no error, and if no byte from the client, then send the Current Data value to the client with the TCP Write function."
        n223 = in-place {
          in-place-border: w597 -> [w602]
          in-place-border: [w601] -> w596
          n224 = in-place-cluster #8(w595) -> ("Clients"=w599:refnum<k5>[])
          n225 = for {
            tunnel: w599 -> [w608] mode=indexing
            shift-right: [w604] -> w601
            shift-left: w602 -> [w603]
            tunnel: [w606] -> w598 mode=indexing if=w605
            w607 = 4  # bytes to read
            n226 = while {
              tunnel: w607 -> [w616]
              tunnel: [w613] -> w605
              shift-right: [w614] -> w606
              shift-left: w608 -> [w618]
              shift-right: [w611] -> w604
              shift-left: w603 -> [w612]
              stop <- w610 stop-if-true
              n227 = TCP Read(connection ID=w618, bytes to read=w616, error in (no error)=w612) -> (connection ID out=w617:refnum<k5>, data out=w615:string, error out=w609:errorcluster)  [unwired: 1 in, 1 out]
              n228 = case shown="에러 없음" w609 {
                selector: w609 -> [w622 w637]
                tunnel: w617 -> [w629 w635]
                tunnel: w615 -> [w630 _]
                tunnel: [w629 w633] -> w614
                tunnel: [w621 w634] -> w613
                tunnel: [w622 w632] -> w611
                tunnel: w609 -> [_ w636]
                tunnel: [w621 w631] -> w610
                frame No Error {
                  w621 = FALSE
                  # "If the client sent data, it is saying that the connection should be closed."
                  # "If the client sent data, it is saying that the connection should be closed."
                  n229 = Unflatten From String(type=cluster{"bx":sgl} {"bx"=0.0}, binary string=w630, byte order (0:big-endian, network order)=T5."little-endian") -> (value=w627:cluster{"bx":sgl})  [unwired: 2 in, 2 out]
                  n230 = Cluster To Array(cluster=w627) -> (array=w624:sgl[])
                  n231 = Greater Or Equal?(x=w624, y=0.5) -> (x >= y?=w620:bool[])
                  n232 = Index Array(array=w620, index=0) -> (element=→"불리언 3":bool)
                }
                frame Error {
                  # "Ignore connection closed and timeout errors"
                  n233 = Unbundle By Name(w637) -> ("code"=w638:i32)
                  n234 = case shown="56" w638 {
                    tunnel: w637 -> [w640 _ _]
                    tunnel: [w640 w643 errorcluster {"status"=FALSE, "code"=0, "source"=""} ("error constant")] -> w632
                    tunnel: w636 -> [_ w643 _]
                    tunnel: w635 -> [_ w642 _]
                    tunnel: [w639 w641 FALSE] -> w634
                    tunnel: [_ w642 _] -> w633
                    tunnel: [w639 w641 TRUE] -> w631
                    frame Default {
                      w639 = FALSE
                      # "Unknown error, pass it through."
                    }
                    frame 56 {
                      w641 = TRUE
                      # "If the TCP Read function timed out, then the connection is still valid, so we can send the current data to the client. Append the string length to the data so the client knows how many bytes to read."
                    }
                    frame 66 {
                      # "The connection was closed, so this client refnum is no longer valid."
                    }
                  }
                }
              }
            }
          }
          n235 = Array Size(array=w598) -> (size(s)=→"# of Connections 4":i32)
          n236 = in-place-cluster #8("Clients"=w598) -> (w594:T1)
        }
      }
      frame "Stop" {
        w647 = TCP_Multiple_Connections_State."Stop"  # (Value Not Used)
        w654 = TRUE  # Stop Loop?
        # "Close all open client connections and the listener connection with TCP Close Connection functions."
        n237 = Unbundle By Name(w653) -> ("Clients"=w651:refnum<k5>[], "Listener"=w648:refnum<k5>)
        n238 = TCP Close Connection(connection ID=w648, error in (no error)=w652) -> (error out=w649:errorcluster)  [unwired: 1 in, 1 out]
        n239 = for {
          shift-right: [w656] -> w650
          shift-left: w649 -> [w657]
          tunnel: w651 -> [w655] mode=indexing
          n240 = TCP Close Connection(connection ID=w655, error in (no error)=w657) -> (error out=w656:errorcluster)  [unwired: 1 in, 1 out]
        }
      }
    }
  }
